vi "timekeeper get time.vi"() -> (0 "time (ns)(g)":fxp<+,64,64>)   [LabVIEW 2011, in "EPS_Timekeeper.lvlib"]
uses:
  <vilib>/addons/Electrical Power/Example Support/PMU/Time Keeper/EPS_Timekeeper.lvlib
  <vilib>/addons/Electrical Power/Example Support/PMU/Time Keeper/timekeeper time (g).vi
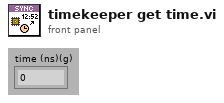
[diagram p1: front panel]
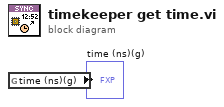
[diagram p0: block diagram]
diagram:
  n1 = global read "timekeeper time (g).vi" "time (ns)(g)"() -> (→"time (ns)(g)":fxp<+,64,64>)
